vi "Set working status.vi"(6 "Enum":enum16{"Set done", "Set working", "Initialize"}(ring), 8 "Error In":errorcluster, 10 "Statuses Array":string[](array[string])=["DONE!", "WORKING", "Initializing"], 11 "reference":refnum<vi>) -> (0 "Error Out":errorcluster)   [LabVIEW 2015]
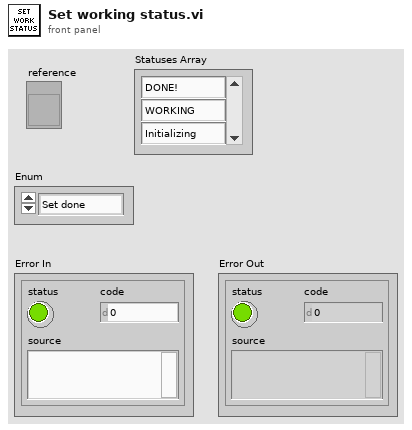
[diagram p1: front panel]
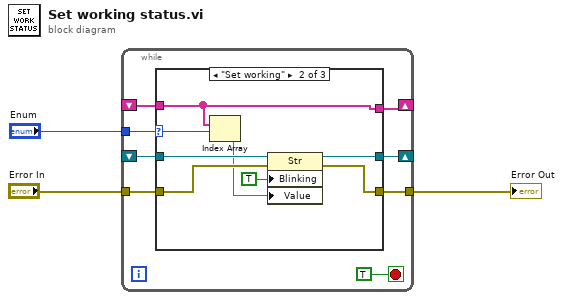
[diagram p0: block diagram]
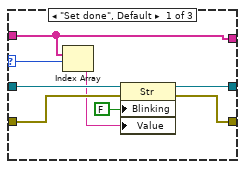
[diagram p2: hidden frame]
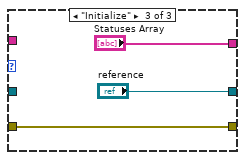
[diagram p3: hidden frame]
diagram:
  n1 = while {
    tunnel: "Enum" -> [w11]
    shift-right: [w10] -> _
    shift-left: _ -> [w9]
    shift-right: [w8] -> _
    shift-left: _ -> [w7]
    tunnel: "Error In" -> [w6]
    tunnel: [w5] -> w1
    stop <- TRUE stop-if-true
    n2 = case shown="\"Set working\"" w11 {
      selector: w11 -> [w19 w27 _]
      tunnel: [w16 w24 "reference"] -> w10
      tunnel: w9 -> [w17 w25 _]
      tunnel: [w18 w26 "Statuses Array"] -> w8
      tunnel: w7 -> [w18 w26 _]
      tunnel: w6 -> [w15 w23 w28]
      tunnel: [w14 w22 w28] -> w5
      frame "Set done", Default {
        n3 = Index Array(array=w18, index=w19) -> (element=w13:string)
        n4 = property on="Property Node" class="Str"(reference=w17, error in=w15, "Blinking"=FALSE, "Value"=w13) -> (reference out=w16:refnum<vi>, error out=w14:errorcluster)
      }
      frame "Set working" {
        n5 = Index Array(array=w26, index=w27) -> (element=w21:string)
        n6 = property on="Property Node" class="Str"(reference=w25, error in=w23, "Blinking"=TRUE, "Value"=w21) -> (reference out=w24:refnum<vi>, error out=w22:errorcluster)
      }
      frame "Initialize" {
      }
    }
  }
  "Error Out" <- w1
